vi "Get Node Info.vi"(8 "error in (no error)":errorcluster, 10 "Active Build Configuration":string, 11 "ZIP Item in":refnum<class "ZIP Item.lvclass">) -> (0 "error out":errorcluster, 1 "Child Nodes":refnum<class "Node.lvclass">[](array[class]), 2 "Label":string)   [LabVIEW 2019, in "ZIP.lvlib" / "ZIP Item.lvclass"]
uses:
  ZIP Item.lvclass
  libs/Solution.lvlibp/Solution/Tree Entry/Node.lvclass
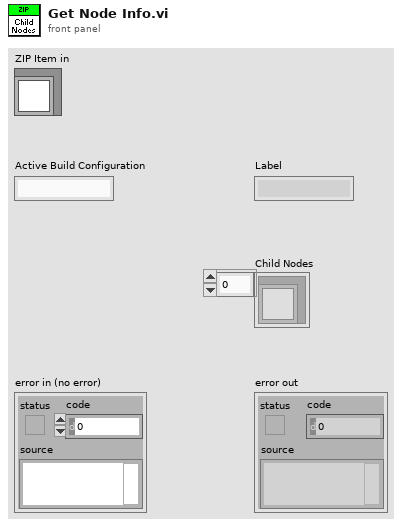
[diagram p1: front panel]
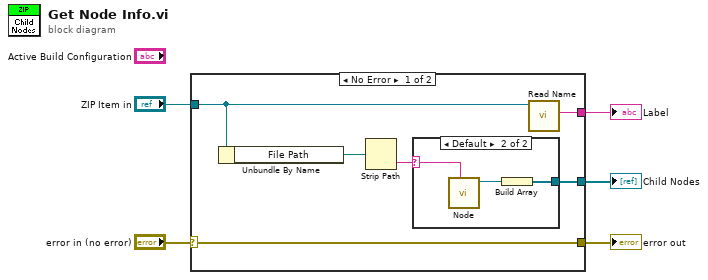
[diagram p0: block diagram]
diagram:
  n1 = case shown="No Error" "error in (no error)" {
    selector: "error in (no error)" -> [w6 w15]
    tunnel: [w11 _] -> w5
    tunnel: [w10 _] -> w4
    tunnel: "ZIP Item in" -> [w9 _]
    tunnel: [w6 w15] -> w2
    frame No Error {
      n2 = Unbundle By Name(w9) -> ("File Path"=w8:path)
      n3 = Strip Path(path=w8) -> (name=w7:string)  [unwired: 1 out]
      n4 = case shown="Default" w7 {
        selector: w7 -> [_ w12]
        tunnel: [_ w13] -> w10
        frame "" {
        }
        frame Default {
          n5 = call "Node.vi"("Name"=w12) -> ("Tree Entry out"=w14:refnum<class "Node.lvclass">)  [unwired: 10 in]
          n6 = Build Array(w14) -> (w13:refnum<class "Node.lvclass">[])
        }
      }
      n7 = call-dynamic "Read Name.vi"("ZIP Item in"=w9) -> ("Name"=w11:string)  [unwired: 10 in]
    }
    frame Error {
    }
  }
  "error out" <- w2
  "Child Nodes" <- w4
  "Label" <- w5
